vi "Receive.vi"(7 "Msg in":refnum<class "Msg.lvclass">, 11 "Teardown State in":refnum<class "Teardown State.lvclass">) -> (5 "Msg out":refnum<class "Msg.lvclass">)   [LabVIEW 2021, in "jettl.lvlib" / "Teardown State.lvclass"]
uses:
  Teardown State.lvclass
  Actor/Msg/Msg.lvclass
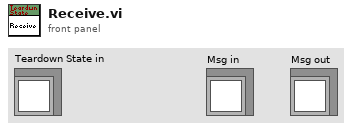
[diagram p1: front panel]
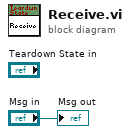
[diagram p0: block diagram]
diagram:
  "Msg out" <- "Msg in"
